vi "Validate_Destinations.vi"(8 "error in (no error)":errorcluster, 11 "AB_DepPackedLibrary in":refnum<class "AB_DepPackedLibrary.lvclass">) -> (0 "error out":errorcluster, 3 "AB_DepPackedLibrary out":refnum<class "AB_DepPackedLibrary.lvclass">)   [LabVIEW 2020, in "AB_DepPackedLibrary.lvclass"]
uses:
  <vilib>/AppBuilder/AB_Classes/DepPackedLib/AB_DepPackedLibrary.lvclass
  e:/builds/penguin/labview/branches/2020/dev/dist/vi.lib/AppBuilder/AB_Classes/Build/AB_Build.lvclass
  <vilib>/AppBuilder/AB_Classes/Build/AB_Build.lvclass
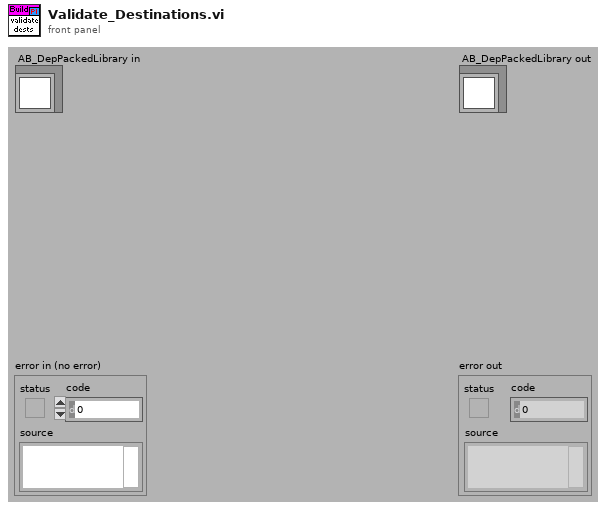
[diagram p1: front panel]
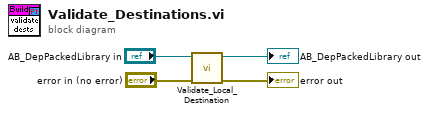
[diagram p0: block diagram]
diagram:
  n1 = call <vilib>:"Validate_Local_Destination.vi"("error in (no error)"="error in (no error)", "AB_Build in"="AB_DepPackedLibrary in") -> ("error out"=→"error out":errorcluster, "AB_Build out"=→"AB_DepPackedLibrary out":refnum<class "AB_DepPackedLibrary.lvclass">)  [unwired: 8 in]
